vi "InTake Set.vi"(0 "InTake":cluster{"TakeBall":dbl, "MoveArm":T1}) -> ()   [LabVIEW 2013]
uses:
  <vilib>/Rock Robotics/WPI/Solenoid/WPI_SolenoidValue.ctl
  <vilib>/Rock Robotics/WPI/Solenoid/WPI_SolenoidSetEnum.vi
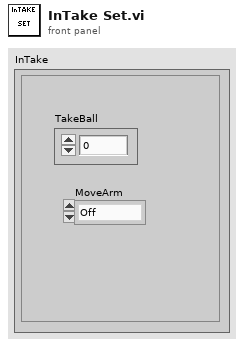
[diagram p1: front panel]
types:
  T1 = typedef "WPI_SolenoidValue.ctl" = enum16{"Off", "On", "Forward", "Reverse"}
  T2 = typedef "WPI_SolenoidDevRef.ctl" = cluster{"DevStatus":errorcluster, "Solenoid Module":T3, "Forward Solenoid Channel":T4, "Reverse Solenoid Channel":T4}
  T3 = typedef "FPGA_TypedefSolenoidModule.ctl" = enum16{"Solenoid Module 1", "Solenoid Module 2"}
  T4 = typedef "WPI_SolenoidChannel.ctl" = enum8{"Solenoid 1", "Solenoid 2", "Solenoid 3", "Solenoid 4", "Solenoid 5", "Solenoid 6", "Solenoid 7", "Solenoid 8", "Invalid"}
  T5 = typedef "WPI_RelayDevRef.ctl" = cluster{"DevStatus":errorcluster, "Relay Channel":T6, "Digital Module":T7, "Relay Direction":T8}
  T6 = typedef "FPGA_DIORelayChannel.ctl" = enum8{"Relay 1", "Relay 2", "Relay 3", "Relay 4", "Relay 5", "Relay 6", "Relay 7", "Relay 8", "Invalid"}
  T7 = typedef "FPGA_TypedefDigitalModule.ctl" = enum16{"Digital Module 1", "Digital Module 2"}
  T8 = typedef "WPI_RelayDirection.ctl" = enum16{"Both directions", "Forward only", "Reverse only"}
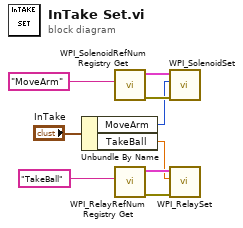
[diagram p0: block diagram]
diagram:
  n1 = Unbundle By Name("InTake") -> ("MoveArm"=w5:T1, "TakeBall"=w1:dbl)
  n2 = call <vilib>:"WPI_SolenoidRefNum Registry Get.vi"("refnum name"="MoveArm") -> ("error out"=w6:errorcluster, "SolenoidDevRef"=w7:T2)  [unwired: 9 in]
  n3 = call <vilib>:"WPI_RelayRefNum Registry Get.vi"("refnum name"="TakeBall") -> ("error out"=w3:errorcluster, "RelayDevRef"=w4:T5)  [unwired: 9 in]
  n4 = call-poly <vilib>:"WPI_SolenoidSet.vi"("error in (no error)"=w6, "Value"=w5, "SolenoidDevRef"=w7) -> ()  [unwired: 7 in, 2 out]
  n5 = call <vilib>:"WPI_RelaySet.vi"("error in (no error)"=w3, "RelayValue"=w1, "RelayDevRef"=w4) -> ()  [unwired: 7 in, 2 out]
